vi "Dictionary to Indicator.vi"(0 "Results (Dictionary)":cluster{"key":string, "value":dbl}[](array[cluster]), 5 "AI Channel":i32=1 max=7 step=1, 11 "error in (no error)":errorcluster) -> (4 "X":dbl, 6 "Y":dbl, 8 "R":dbl, 10 "Theta":dbl, 15 "error out":errorcluster)   [LabVIEW 2019, in "Instrument.Lockin.lvlib" / "Instrument UI.Lockin.lvclass"]
uses:
  Instrument UI.Lockin.lvclass
  Instrument.Lockin/Typedefs/Results Type--Enum.ctl
  Instrument.Lockin/Instrument.Lockin.lvclass
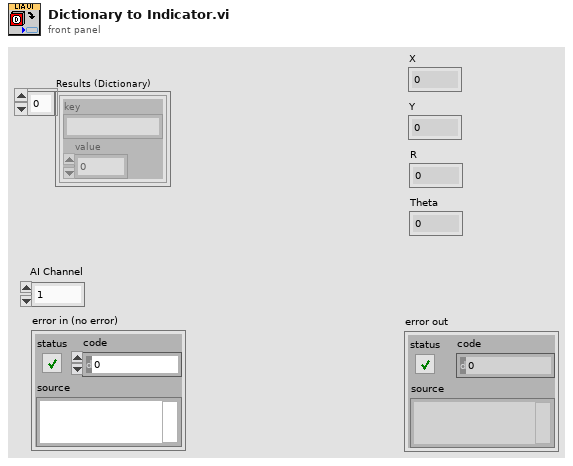
[diagram p1: front panel]
types:
  T1 = typedef "Instrument.Lockin.lvlib/Instrument.Lockin.lvclass/Results Type--Enum.ctl" = enum16{"X", "Y", "R", "Theta", "Mean"}
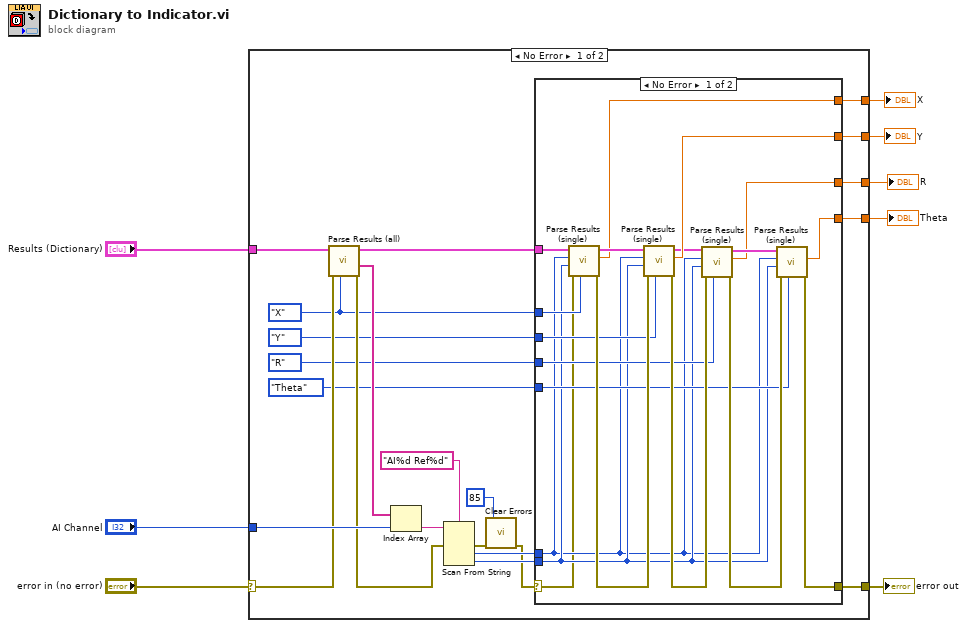
[diagram p0: block diagram]
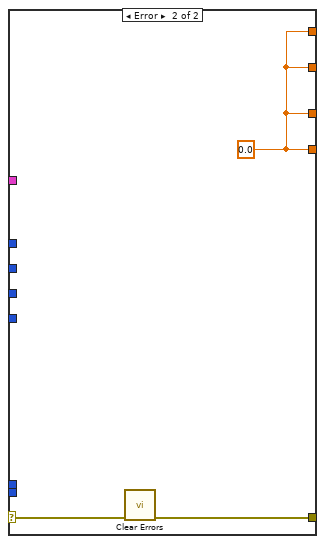
[diagram p2: hidden frame]
diagram:
  n1 = case shown="No Error" "error in (no error)" {
    selector: "error in (no error)" -> [w19 w53]
    tunnel: "Results (Dictionary)" -> [w30 _]
    tunnel: "AI Channel" -> [w26 _]
    tunnel: [w27 _] -> w6
    tunnel: [w28 _] -> w5
    tunnel: [w17 w53] -> w3
    tunnel: [w11 _] -> w1
    tunnel: [w10 _] -> w2
    frame No Error {
      w18 = Results_Type--Enum."X" ("Type")
      n2 = call "Parse Results (all).vi"("Type"=w18, "error in (no error)"=w19, "Results (Dictionary)"=w30) -> ("error out"=w24:errorcluster, "Names"=w23:string[], "Results (Dictionary)"=w29:cluster{"key":string, "value":dbl}[])  [unwired: 5 in, 1 out]
      n3 = Index Array(array=w23, index=w26) -> (element=w25:string)
      n4 = Scan From String(format string="AI%d Ref%d", input string=w25, error in=w24) -> (error out=w21:errorcluster, output 1=w12:i32, output 2=w13:i32)  [unwired: 3 in, 2 out]
      n5 = call <vilib>:"Clear Errors.vi"("error in (no error)"=w21, "specific error code to clear (0: all)"=85) -> ("error out"=w9:errorcluster)  [unwired: 4 in, 1 out]
      n6 = case shown="No Error" w9 {
        selector: w9 -> [w31 w51]
        tunnel: w29 -> [w49 _]
        tunnel: [w47 w52] -> w28
        tunnel: [w46 w52] -> w27
        tunnel: w18 -> [w44 _]
        tunnel: [w40 w50] -> w17
        tunnel: Results_Type--Enum."Y" ("Type") -> [w39 _]
        tunnel: Results_Type--Enum."R" ("Type") -> [w38 _]
        tunnel: Results_Type--Enum."Theta" ("Type") -> [w36 _]
        tunnel: w13 -> [w35 _]
        tunnel: w12 -> [w34 _]
        tunnel: [w33 w52] -> w11
        tunnel: [w32 w52] -> w10
        frame No Error {
          n7 = call "Parse Results (single).vi"("Type"=w44, "error in (no error)"=w31, "Reference Channel"=w35, "AI Channel"=w34, "Results (Dictionary)"=w49) -> ("error out"=w45:errorcluster, "Data"=w46:dbl, "Results (Dictionary)"=w48:cluster{"key":string, "value":dbl}[])  [unwired: 3 in, 1 out]
          n8 = call "Parse Results (single).vi"("Type"=w39, "error in (no error)"=w45, "Reference Channel"=w35, "AI Channel"=w34, "Results (Dictionary)"=w48) -> ("error out"=w42:errorcluster, "Data"=w47:dbl, "Results (Dictionary)"=w37:cluster{"key":string, "value":dbl}[])  [unwired: 3 in, 1 out]
          n9 = call "Parse Results (single).vi"("Type"=w38, "error in (no error)"=w42, "Reference Channel"=w35, "AI Channel"=w34, "Results (Dictionary)"=w37) -> ("error out"=w41:errorcluster, "Data"=w33:dbl, "Results (Dictionary)"=w43:cluster{"key":string, "value":dbl}[])  [unwired: 3 in, 1 out]
          n10 = call "Parse Results (single).vi"("Type"=w36, "error in (no error)"=w41, "Reference Channel"=w35, "AI Channel"=w34, "Results (Dictionary)"=w43) -> ("error out"=w40:errorcluster, "Data"=w32:dbl)  [unwired: 3 in, 2 out]
        }
        frame Error {
          w52 = 0.0 ("Data")
          n11 = call <vilib>:"Clear Errors.vi"("error in (no error)"=w51) -> ("error out"=w50:errorcluster)  [unwired: 5 in, 1 out]
        }
      }
    }
    frame Error {
    }
  }
  "X" <- w6
  "Y" <- w5
  "error out" <- w3
  "R" <- w1
  "Theta" <- w2
